vi "Handle Exception.vi"(7 "Processing In":refnum<class "Processing.lvclass">, 8 "error in (no error)":errorcluster, 11 "SSE Handler in":refnum<class "SSE Handler.lvclass">) -> (0 "error out":errorcluster, 5 "Processing":refnum<class "Processing.lvclass">)   [LabVIEW 2020, in "HTTP Server.lvlib" / "SSE Handler.lvclass"]
uses:
  SSE Handler.lvclass
  SSE Handler.lvclass/SSE Handler.ctl
  Processing/Processing.lvclass
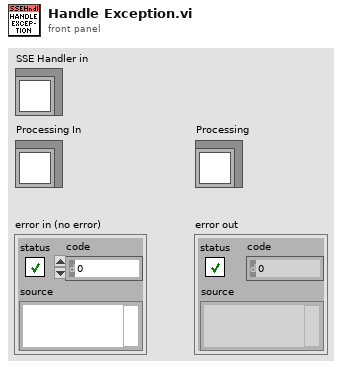
[diagram p1: front panel]
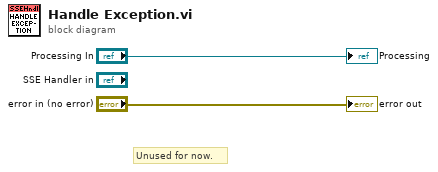
[diagram p0: block diagram]
diagram:
  # "Unused for now."
  "error out" <- "error in (no error)"
  "Processing" <- "Processing In"
